vi "launchee.vi"() -> ()   [LabVIEW 2014]
panel:
  out "number (0 to 1)":dbl
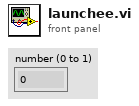
[diagram p1: front panel]
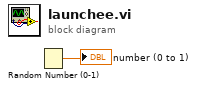
[diagram p0: block diagram]
diagram:
  n1 = Random Number (0-1)() -> (number: 0 to 1=→"number (0 to 1)":dbl)
